vi "Initialize_main_SubVI.vi"() -> (0 "output cluster":T26 {"A/SPI - LiDAR"."SPI Configuration"."Frame Length" min=1 max=16})   [LabVIEW 2018]
uses:
  <vilib>/myRIO/Instrument Drivers/Onboard IO/DIO/typedefs/DIO Reference.ctl
  <vilib>/myRIO/Common/Instrument Driver Framework/Utilities/typedefs/myRIO Generic Hardware Reference.ctl
  <vilib>/myRIO/Common/Instrument Driver Framework/Utilities/typedefs/Hardware Version Enum.ctl
  <vilib>/myRIO/Common/Instrument Driver Framework/Utilities/typedefs/myRIO v1.0 Reference.ctl
  <vilib>/myRIO/Common/Instrument Driver Framework/Utilities/typedefs/Generic FPGA Reference.ctl
  <vilib>/myRIO/Common/Instrument Driver Framework/myRIO v1.0/DIO/typedefs/DIO Channels List.ctl
  <vilib>/myRIO/Common/Instrument Driver Framework/myRIO v1.0/DIO/typedefs/DIO Channels Enum.ctl
  <vilib>/myRIO/Instrument Drivers/Onboard IO/PWM/typedefs/PWM Reference.ctl
  <vilib>/myRIO/Common/Instrument Driver Framework/myRIO v1.0/PWM/typedefs/PWM Channels Enum.ctl
  <vilib>/myRIO/Instrument Drivers/Onboard IO/PWM/typedefs/PWM Configuration.ctl
  <vilib>/myRIO/Instrument Drivers/Onboard Devices/Accelerometer/typedefs/Accelerometer Reference.ctl
  <vilib>/myRIO/Common/Instrument Driver Framework/myRIO v1.0/Accelerometer/typedefs/Accelerometer Channels List.ctl
  <vilib>/myRIO/Common/Instrument Driver Framework/myRIO v1.0/Accelerometer/typedefs/Accelerometer Channels Enum.ctl
  <vilib>/myRIO/Instrument Drivers/Onboard IO/AI/typedefs/AI Reference.ctl
  <vilib>/myRIO/Common/Instrument Driver Framework/myRIO v1.0/AI/typedefs/AI Channels List.ctl
  <vilib>/myRIO/Common/Instrument Driver Framework/myRIO v1.0/AI/typedefs/AI Channels Enum.ctl
  <vilib>/myRIO/Common/Instrument Driver Framework/Utilities/typedefs/Analog Scaling Constants List.ctl
  <vilib>/myRIO/Common/Instrument Driver Framework/Utilities/typedefs/Analog Scaling Constants.ctl
  <vilib>/myRIO/Instrument Drivers/Onboard IO/SPI/typedefs/SPI Reference.ctl
  <vilib>/myRIO/Common/Instrument Driver Framework/myRIO v1.0/SPI/typedefs/SPI Channels Enum.ctl
  <vilib>/myRIO/Instrument Drivers/Onboard IO/SPI/typedefs/SPI Configuration.ctl
  <vilib>/myRIO/Common/Instrument Driver Framework/myRIO v1.0/SPI/typedefs/SPI Clock Phase.ctl
  <vilib>/myRIO/Common/Instrument Driver Framework/myRIO v1.0/SPI/typedefs/SPI Clock Polarity.ctl
  <vilib>/myRIO/Common/Instrument Driver Framework/myRIO v1.0/SPI/typedefs/SPI Data Direction.ctl
  <vilib>/myRIO/Common/Instrument Driver Framework/myRIO v1.0/SPI/typedefs/SPI Frame Length.ctl
  <vilib>/userdefined/High Color/nirio_resource_hc.ctl
  <vilib>/myRIO/Common/Instrument Driver Framework/myRIO v1.0/SPI/vis/myRIO v1.1 Open SPI.vi
  <vilib>/myRIO/Common/Instrument Driver Framework/myRIO v1.0/AI/vis/myRIO v1.1 Open AI.vi
  <vilib>/myRIO/Common/Instrument Driver Framework/myRIO v1.0/PWM/vis/myRIO v1.1 Open PWM.vi
  <vilib>/myRIO/Common/Instrument Driver Framework/myRIO v1.0/DIO/vis/myRIO v1.1 Open DIO.vi
  <vilib>/myRIO/Common/Instrument Driver Framework/myRIO v1.0/Accelerometer/vis/myRIO v1.1 Open Accelerometer.vi
  <vilib>/myRIO/Common/Instrument Driver Framework/Utilities/vis/Validate Channels.vi
  <vilib>/myRIO/Common/Instrument Driver Framework/myRIO v1.0/SPI/vis/myRIO v1.0 Reserve SPI.vi
  <vilib>/myRIO/Common/Instrument Driver Framework/myRIO v1.0/AI/vis/myRIO v1.0 Reserve AI.vi
  <vilib>/myRIO/Common/Instrument Driver Framework/myRIO v1.0/PWM/vis/myRIO v1.0 Reserve PWM.vi
  <vilib>/myRIO/Common/Instrument Driver Framework/myRIO v1.0/DIO/vis/myRIO v1.0 Reserve DIO.vi
  <vilib>/myRIO/Common/Instrument Driver Framework/myRIO v1.0/Accelerometer/vis/myRIO v1.0 Reserve Accelerometer.vi
  <vilib>/myRIO/Common/Instrument Driver Framework/myRIO v1.0/SPI/vis/myRIO v1.0 Build MUX Configuration SPI.vi
  <vilib>/myRIO/Common/Instrument Driver Framework/myRIO v1.0/Resource Manager/vis/myRIO v1.0 Reserve Channel List.vi
  <vilib>/myRIO/Common/Instrument Driver Framework/myRIO v1.0/AI/vis/myRIO v1.0 Build MUX Configuration AI.vi
  <vilib>/myRIO/Common/Instrument Driver Framework/myRIO v1.0/PWM/vis/myRIO v1.0 Build MUX Configuration PWM.vi
  <vilib>/myRIO/Common/Instrument Driver Framework/myRIO v1.0/DIO/vis/myRIO v1.0 Build MUX Configuration DIO.vi
  <vilib>/myRIO/Common/Instrument Driver Framework/myRIO v1.0/Accelerometer/vis/myRIO v1.0 Build MUX Configuration Accelerometer.vi
  <vilib>/myRIO/Common/Instrument Driver Framework/myRIO v1.0/Resource Manager/vis/myRIO v1.0 Create Configuration List.vi
  <vilib>/myRIO/Common/Instrument Driver Framework/myRIO v1.0/Resource Manager/vis/myRIO v1.0 Reserve Channel.vi
  <vilib>/myRIO/Common/Instrument Driver Framework/myRIO v1.0/Resource Manager/vis/myRIO v1.0 Unreserve Channel.vi
  <vilib>/myRIO/Common/Instrument Driver Framework/myRIO v1.0/Resource Manager/vis/myRIO v1.0 Build Mutex Name.vi
  <vilib>/Instr/_visa.llb/VISA Configure Serial Port (Instr).vi
  <vilib>/Utility/VariantDataType/GetNumericInfo.vi
  <vilib>/Utility/error.llb/Error Cluster From Error Code.vi
  <vilib>/myRIO/Common/Instrument Driver Framework/myRIO v1.0/myRIO v1.1 Open.vi
  <vilib>/myRIO/Common/Instrument Driver Framework/Utilities/vis/IO Manager.vi
  <vilib>/myRIO/Common/Instrument Driver Framework/Utilities/vis/Configuration Manager.vi
  <vilib>/myRIO/Common/Instrument Driver Framework/myRIO v1.0/Resource Manager/vis/myRIO v1.0 Configure IO.vi
  <vilib>/myRIO/Common/Instrument Driver Framework/myRIO v1.0/myRIO v1.0 Close.vi
  <vilib>/myRIO/Common/Instrument Driver Framework/myRIO v1.0/AI/vis/myRIO v1.0 Get Scaling Constants AI.vi
  <vilib>/myRIO/Common/Instrument Driver Framework/myRIO v1.0/Accelerometer/vis/myRIO v1.0 Get Scaling Constant Accelerometer.vi
  <vilib>/myRIO/Instrument Drivers/Onboard IO/PWM/vis/myRIO PWM Open.xnode
  <vilib>/myRIO/Instrument Drivers/Onboard IO/AI/vis/myRIO AI Open.xnode
  <vilib>/myRIO/Instrument Drivers/Onboard IO/DIO/vis/myRIO DIO Open.xnode
  <vilib>/myRIO/Instrument Drivers/Onboard Devices/Accelerometer/vis/myRIO Accelerometer Open.xnode
  <vilib>/myRIO/Instrument Drivers/Onboard IO/SPI/vis/myRIO SPI Open.xnode
  <vilib>/myRIO/Instrument Drivers/Onboard IO/DIO/DIO.lvlib
  <vilib>/myRIO/Instrument Drivers/Onboard IO/PWM/PWM.lvlib
  <vilib>/myRIO/Instrument Drivers/Onboard IO/AI/AI.lvlib
  <vilib>/myRIO/Instrument Drivers/Onboard Devices/Accelerometer/Accelerometer.lvlib
  <vilib>/myRIO/Instrument Drivers/Onboard IO/SPI/SPI.lvlib
panel:
  # "B/DIO0-Dir"
  # "DIR"
  # "B/DIO1-Enable for 1st Stepper"
  # "EN-1"
  # "B/DIO2-Enable for 2nd Stepper"
  # "EN-2"
  # "B/DIO3-Enable for 3nd Stepper"
  # "EN-3"
  # "B/DIO4-Endstop for 1st Stepper - Top"
  # "END-1-T"
  # "B/DIO11-Endstop for 1st Stepper - Bottom"
  # "END-1-B"
  # "B/DIO12-Endstop for 2nd Stepper - Top"
  # "END-2-T"
  # "B/DIO13-Endstop for 2nd Stepper - Bottom"
  # "END-2-B"
  # "B/DIO14-Endstop for 3rd Stepper - Top"
  # "END-3-T"
  # "B/DIO15-Endstop for 3rd Stepper - Bottom"
  # "END-3-B"
  # "Cooler"
  # "A/DIO0-Cooler"
  # "A/DIO1-Beacon drop (dio1)"
  # "Beacon drop"
  # "A/DIO2-Beacon drop (dio0)"
  # "Beacon drop"
  # "A/DIO3-QuickRelease (dio1)"
  # "QuickRelease"
  # "A/DIO4-QuickRelease (dio0)"
  # "QuickRelease"
  # "A/DIO11 - LiDAR Case selector"
  # "LiDAR CS"
  # "B/DIO8 - B_PWM0-Motor - Stepper"
  # "PWM-Step"
  # "B/DIO9 - B_PWM1- Drill motor"
  # "PWM-Drill"
  # "A/DIO8 - A_PWM0 - Servo_Roll"
  # "Gimbal_ROLL"
  # "A/DIO9 - A_PWM1 - Servo_Yaw"
  # "Gimbal_YAW"
  # "Accelerometer - X-axis"
  # "X-axis"
  # "Accelerometer - X-axis"
  # "Y-axis"
  # "B/AI0 - PWM from drone F3"
  # "Drone - F3 - Grounded"
  # "B/AI1 - PWM from drone F4"
  # "Drone - F4 - Drill gear"
  # "B/AI2 - PWM from drone F5"
  # "Drone - F5 - Beacon drop"
  # "B/AI3 - PWM from drone F6"
  # "Drone - F6 - Boost"
  # "A/AI0 - PWM from drone F8"
  # "Drone - F8 - Stepper"
  # "A/AI1 - Beacon Wiper"
  # "A/AI2 - QuickRelease Wiper"
  # "A/AI3 - Drill drawn current"
  # "A/SPI - LiDAR Distance measurement"
  # "B/UART - XBee Communication"
  # "A/UART - A3 GPS Coordinates"
  # "RIO - LEDs"
  # "RIO - LEDs"
types:
  T1 = typedef "DIO.lvlib/DIO Reference.ctl" = cluster{"myRIO Reference":T2, "DIO Channels List":T6}
  T2 = typedef "myRIO Generic Hardware Reference.ctl" = cluster{"myRIO Model":T3, "myRIO Hardware Reference":T4}
  T3 = typedef "Hardware Version Enum.ctl" = enum16{"Unknown", "myRIO-1900", "myRIO-1950", "roboRIO", "NI ELVIS RIO CM", "ELVIS III"}
  T4 = typedef "myRIO v1.0 Reference.ctl" = cluster{"Generic FPGA Reference":T5, "Allow multiple opens":bool}
  T5 = typedef "Generic FPGA Reference.ctl" = refnum<k20>
  T6 = typedef "DIO Channels List.ctl" = T7[]
  T7 = typedef "DIO Channels Enum.ctl" = enum16{"Not Connected", "C/DIO0", "C/DIO1", "C/DIO2", "C/DIO3", "C/DIO4", "C/DIO5", "C/DIO6", "C/DIO7", "A/DIO0", "A/DIO1", "A/DIO2", "A/DIO3", "A/DIO4", "A/DIO5", "A/DIO6", "A/DIO7", "A/DIO8", "A/DIO9", "A/DIO10", "A/DIO11", "A/DIO12", "A/DIO13", "A/DIO14", "A/DIO15", "A/DIO16", "A/DIO17", "A/DIO18", "A/DIO19", "B/DIO0", "B/DIO1", "B/DIO2", "B/DIO3", "B/DIO4", "B/DIO5", "B/DIO6", "B/DIO7", "B/DIO8", "B/DIO9", "B/DIO10", "B/DIO11", "B/DIO12", "B/DIO13", "B/DIO14", "B/DIO15", "B/DIO16", "B/DIO17", "B/DIO18", "B/DIO19", "LED0", "LED1", "LED2", "LED3", "Button0", "DIO/DIO0", "DIO/DIO1", "DIO/DIO2", "DIO/DIO3", "DIO/DIO4", "DIO/DIO5", "DIO/DIO6", "DIO/DIO7", "DIO/DIO8", "DIO/DIO9", "SPI/CS0", "SPI/CS1", "SPI/CS2", "SPI/CS3", "LED RADIO (Green)", "LED RADIO (Red)", "LED COMM (Green)", "LED COMM (Red)", "LED MODE (Green)", "LED MODE (Red)"}
  T8 = typedef "PWM.lvlib/PWM Reference.ctl" = cluster{"myRIO Reference":T2, "PWM Channels Enum":T9, "PWM Configuration":T10}
  T9 = typedef "PWM Channels Enum.ctl" = enum16{"Not Connected", "C/PWM0", "C/PWM1", "A/PWM0", "A/PWM1", "A/PWM2", "A/PWM3", "A/PWM4", "A/PWM5", "A/PWM6", "A/PWM7", "A/PWM8", "A/PWM9", "A/PWM10", "A/PWM11", "A/PWM12", "A/PWM13", "A/PWM14", "A/PWM15", "A/PWM16", "A/PWM17", "A/PWM18", "A/PWM19", "B/PWM0", "B/PWM1", "B/PWM2", "B/PWM3", "B/PWM4", "B/PWM5", "B/PWM6", "B/PWM7", "B/PWM8", "B/PWM9", "B/PWM10", "B/PWM11", "B/PWM12", "B/PWM13", "B/PWM14", "B/PWM15", "B/PWM16", "B/PWM17", "B/PWM18", "B/PWM19", "PWM/PWM0", "PWM/PWM1", "PWM/PWM2", "PWM/PWM3", "PWM/PWM4", "PWM/PWM5", "PWM/PWM6", "PWM/PWM7", "PWM/PWM8", "PWM/PWM9"}
  T10 = typedef "PWM.lvlib/PWM Configuration.ctl" = cluster{"Frequency":dbl, "Duty Cycle":dbl}
  T11 = typedef "Accelerometer.lvlib/Accelerometer Reference.ctl" = cluster{"myRIO Reference":T2, "Accelerometer Channels List":T12, "LSB Weight":dbl}
  T12 = typedef "Accelerometer Channels List.ctl" = T13[]
  T13 = typedef "Accelerometer Channels Enum.ctl" = enum16{"Not Connected", "X-Axis", "Y-Axis", "Z-Axis"}
  T14 = typedef "AI.lvlib/AI Reference.ctl" = cluster{"myRIO Reference":T2, "AI Channels List":T15, "AI Scaling Constants List":T17}
  T15 = typedef "AI Channels List.ctl" = T16[]
  T16 = typedef "AI Channels Enum.ctl" = enum16{"Not Connected", "AudioIn/Left", "AudioIn/Right", "C/AI0", "C/AI1", "A/AI0", "A/AI1", "A/AI2", "A/AI3", "A/AI4", "A/AI5", "A/AI6", "A/AI7", "B/AI0", "B/AI1", "B/AI2", "B/AI3", "B/AI4", "B/AI5", "B/AI6", "B/AI7", "AI/AI0", "AI/AI1", "AI/AI2", "AI/AI3", "A/AI0 (DIFF)", "A/AI1 (DIFF)", "A/AI2 (DIFF)", "A/AI3 (DIFF)", "B/AI0 (DIFF)", "B/AI1 (DIFF)", "B/AI2 (DIFF)", "B/AI3 (DIFF)"}
  T17 = typedef "Analog Scaling Constants List.ctl" = T18[]
  T18 = typedef "Analog Scaling Constants.ctl" = cluster{"LSB Weight (Volts)":dbl, "Offset (Volts)":dbl, "Signed?":bool}
  T19 = typedef "SPI.lvlib/SPI Reference.ctl" = cluster{"myRIO Reference":T2, "SPI Channels Enum":T20, "SPI Configuration":T21}
  T20 = typedef "SPI Channels Enum.ctl" = enum16{"Not Connected", "A/SPI", "B/SPI", "SPI/SPI"}
  T21 = typedef "SPI.lvlib/SPI Configuration.ctl" = cluster{"Frequency [Hz]":dbl, "Clock Phase":T22, "Clock Polarity":T23, "Data Direction":T24, "Frame Length":T25}
  T22 = typedef "SPI Clock Phase.ctl" = enum8{"Leading", "Trailing"}
  T23 = typedef "SPI Clock Polarity.ctl" = enum8{"Low", "High"}
  T24 = typedef "SPI Data Direction.ctl" = enum8{"Most significant bit first", "Least significant bit first"}
  T25 = typedef "SPI Frame Length.ctl" = u8
  T26 = cluster{"B/DIO0 - Stepper Direction":T1, "B/DIO1 - Stepper1 Enable":T1, "B/DIO2 - Stepper2 Enable":T1, "B/DIO3 - Stepper3 Enable":T1, "B/DIO4 - Endstop Stepper1 Top":T1, "B/DIO11 - Endstop Stepper1 Bund":T1, "B/DIO12 - Endstop Stepper2 Top":T1, "B/DIO13 - Endstop Stepper2 Bund":T1, "B/DIO14 - Endstop Stepper3 Top":T1, "B/DIO15 - Endstop Stepper3 Bund":T1, "A/DIO0 - Cooler":T1, "A/DIO1 - Beacon drop (dio1)":T1, "A/DIO2 - Beacon drop (dio0)":T1, "A/DIO3 - QuickRelease (dio1)":T1, "A/DIO4 - QuickRelease (dio0)":T1, "A/DIO11 - LiDAR SPI CS":T1, "B/PWM0 - Stepper":T8, "B/PWM1 - Drill":T8, "A/PWM0 - Servo_Roll":T8, "A/PWM1 - Servo_Yaw":T8, "Acc. X-axis":T11, "Acc. Y-axis":T11, "B/AI0 - Drone Grounded F3":T14, "B/AI1 - Drone Drill Gear F4":T14, "B/AI2 - Beacon Drop F5":T14, "B/AI3 - Drone Drill Boost F6":T14, "A/AI0 - Drone Stepper F8":T14, "A/AI1 - Beacon Wiper":T14, "A/AI2 - QuickRelease Wiper":T14, "A/AI3 - Drill Current":T14, "A/SPI - LiDAR":T19, "B/UART - XBee":refnum<visa-resource-name>, "A/UART - A3 GPS":refnum<visa-resource-name>, "RIO Flashing LEDs":T1}
  T27 = cluster{"DIO Ref Out":T1, "DIO Ref Out":T1, "DIO Ref Out":T1, "DIO Ref Out":T1, "DIO Ref Out":T1, "DIO Ref Out":T1, "DIO Ref Out":T1, "DIO Ref Out":T1, "DIO Ref Out":T1, "DIO Ref Out":T1, "DIO Ref Out":T1, "DIO Ref Out":T1, "DIO Ref Out":T1, "DIO Ref Out":T1, "DIO Ref Out":T1, "DIO Ref Out":T1, "PWM Ref Out":T8, "PWM Ref Out":T8, "PWM Ref Out":T8, "PWM Ref Out":T8, "Accelerometer Ref Out":T11, "Accelerometer Ref Out":T11, "AI Ref Out":T14, "AI Ref Out":T14, "AI Ref Out":T14, "AI Ref Out":T14, "AI Ref Out":T14, "AI Ref Out":T14, "AI Ref Out":T14, "AI Ref Out":T14, "SPI Ref Out":T19, "VISA resource name out":refnum<visa-resource-name>, "VISA resource name out":refnum<visa-resource-name>, "DIO Ref Out":T1}
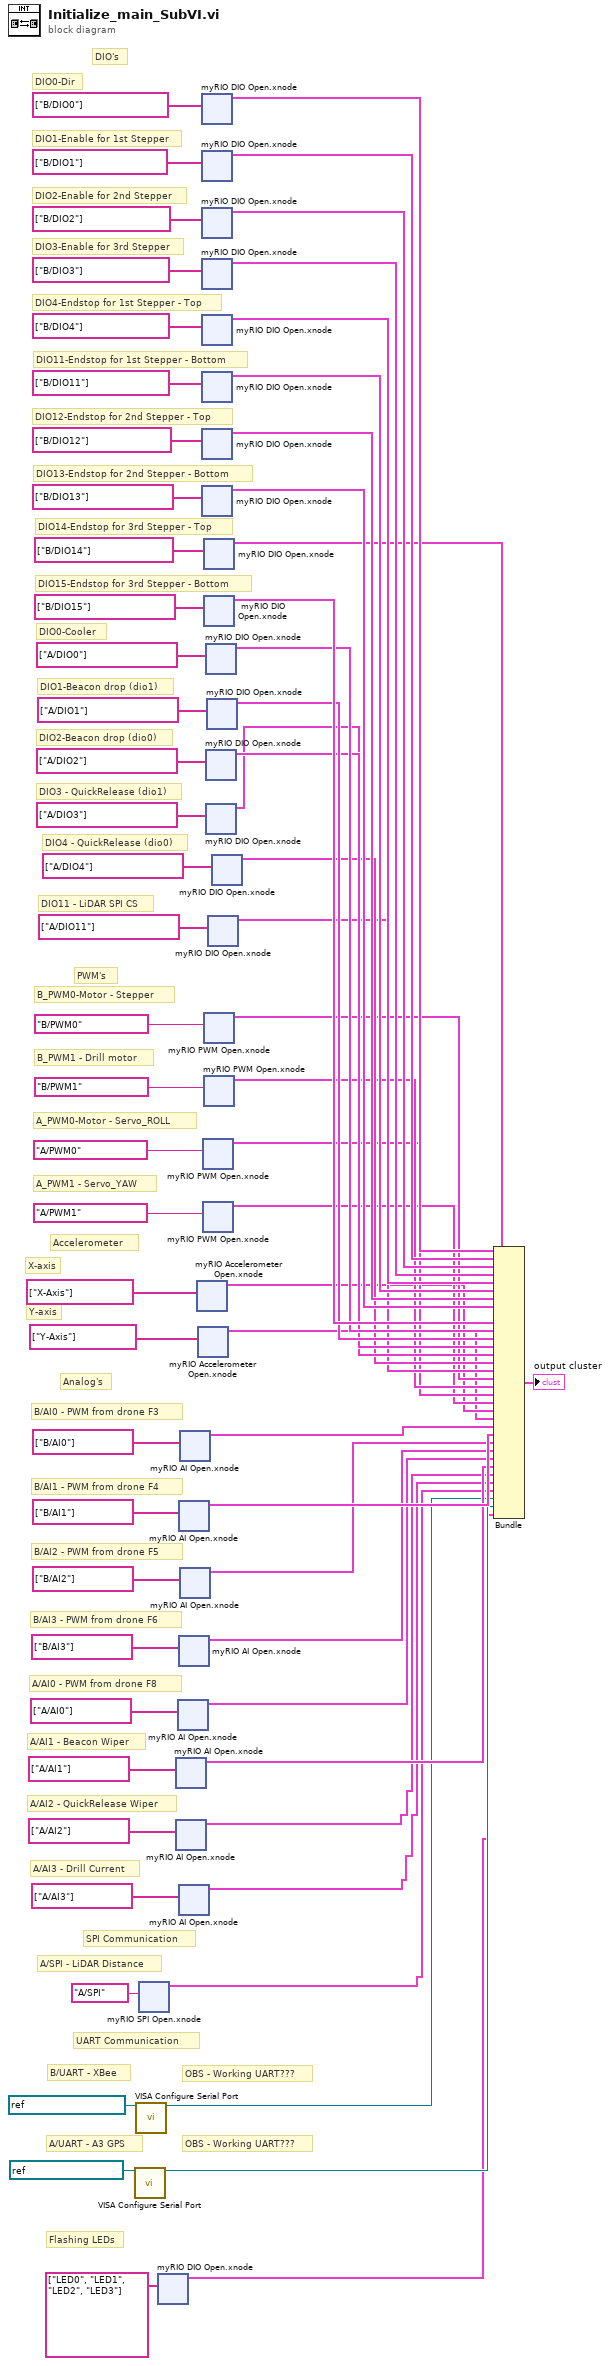
[diagram p0: block diagram]
diagram:
  # "OBS - Working UART???"
  # "OBS - Working UART???"
  # "Flashing LEDs"
  # "A/UART - A3 GPS"
  # "B/UART - XBee"
  # "A/SPI - LiDAR Distance"
  # "UART Communication"
  # "SPI Communication"
  # "A/AI3 - Drill Current"
  # "A/AI2 - QuickRelease Wiper"
  # "A/AI1 - Beacon Wiper"
  # "A_PWM1 - Servo_YAW"
  # "A_PWM0-Motor - Servo_ROLL"
  # "DIO11 - LiDAR SPI CS"
  # "DIO4 - QuickRelease (dio0)"
  # "DIO3 - QuickRelease (dio1)"
  # "DIO2-Beacon drop (dio0)"
  # "DIO1-Beacon drop (dio1)"
  # "Y-axis"
  # "DIO0-Cooler"
  # "A/AI0 - PWM from drone F8"
  # "B/AI3 - PWM from drone F6"
  # "DIO15-Endstop for 3rd Stepper - Bottom"
  # "DIO14-Endstop for 3rd Stepper - Top"
  # "DIO13-Endstop for 2nd Stepper - Bottom"
  # "DIO12-Endstop for 2nd Stepper - Top"
  # "DIO11-Endstop for 1st Stepper - Bottom"
  # "DIO4-Endstop for 1st Stepper - Top"
  # "Accelerometer"
  # "X-axis"
  # "DIO3-Enable for 3rd Stepper"
  # "DIO2-Enable for 2nd Stepper"
  # "DIO1-Enable for 1st Stepper"
  # "DIO0-Dir"
  # "Analog's"
  # "B/AI2 - PWM from drone F5"
  # "B/AI1 - PWM from drone F4"
  # "B/AI0 - PWM from drone F3"
  # "B_PWM1 - Drill motor"
  # "B_PWM0-Motor - Stepper"
  # "PWM's"
  # "DIO's"
  n1 = call-poly "VISA Configure Serial Port"("VISA resource name"=refnum<visa-resource-name> "ASRL1::INSTR") -> ("VISA resource name out"=w3:refnum<visa-resource-name>)  [unwired: 13 in, 1 out]
  n2 = call-poly "VISA Configure Serial Port"("VISA resource name"=refnum<visa-resource-name> "ASRL2::INSTR") -> ("VISA resource name out"=w4:refnum<visa-resource-name>)  [unwired: 13 in, 1 out]
  n3 = xnode "myRIO SPI Open.xnode"("Channel Name"=tag "A/SPI") -> ("SPI Ref Out"=w7:T19)  [unwired: 2 in, 1 out]
  n4 = xnode "myRIO DIO Open.xnode"("Channel Names"=tag[] ["LED0", "LED1", "LED2", "LED3"]) -> ("DIO Ref Out"=w2:T1)  [unwired: 2 in, 1 out]
  n5 = xnode "myRIO AI Open.xnode"("Channel Names"=tag[] ["A/AI1"]) -> ("AI Ref Out"=w11:T14)  [unwired: 2 in, 1 out]
  n6 = xnode "myRIO AI Open.xnode"("Channel Names"=tag[] ["A/AI2"]) -> ("AI Ref Out"=w10:T14)  [unwired: 2 in, 1 out]
  n7 = xnode "myRIO AI Open.xnode"("Channel Names"=tag[] ["A/AI0"]) -> ("AI Ref Out"=w12:T14)  [unwired: 2 in, 1 out]
  n8 = xnode "myRIO AI Open.xnode"("Channel Names"=tag[] ["B/AI1"]) -> ("AI Ref Out"=w15:T14)  [unwired: 2 in, 1 out]
  n9 = xnode "myRIO AI Open.xnode"("Channel Names"=tag[] ["B/AI3"]) -> ("AI Ref Out"=w13:T14)  [unwired: 2 in, 1 out]
  n10 = xnode "myRIO AI Open.xnode"("Channel Names"=tag[] ["A/AI3"]) -> ("AI Ref Out"=w9:T14)  [unwired: 2 in, 1 out]
  n11 = xnode "myRIO AI Open.xnode"("Channel Names"=tag[] ["B/AI0"]) -> ("AI Ref Out"=w16:T14)  [unwired: 2 in, 1 out]
  n12 = xnode "myRIO AI Open.xnode"("Channel Names"=tag[] ["B/AI2"]) -> ("AI Ref Out"=w14:T14)  [unwired: 2 in, 1 out]
  n13 = xnode "myRIO Accelerometer Open.xnode"("Channel Names"=tag[] ["X-Axis"]) -> ("Accelerometer Ref Out"=w21:T11)  [unwired: 2 in, 1 out]
  n14 = xnode "myRIO Accelerometer Open.xnode"("Channel Names"=tag[] ["Y-Axis"]) -> ("Accelerometer Ref Out"=w20:T11)  [unwired: 2 in, 1 out]
  n15 = xnode "myRIO DIO Open.xnode"("Channel Names"=tag[] ["B/DIO0"]) -> ("DIO Ref Out"=w53:T1)  [unwired: 2 in, 1 out]
  n16 = xnode "myRIO DIO Open.xnode"("Channel Names"=tag[] ["B/DIO1"]) -> ("DIO Ref Out"=w52:T1)  [unwired: 2 in, 1 out]
  n17 = xnode "myRIO DIO Open.xnode"("Channel Names"=tag[] ["B/DIO2"]) -> ("DIO Ref Out"=w51:T1)  [unwired: 2 in, 1 out]
  n18 = xnode "myRIO DIO Open.xnode"("Channel Names"=tag[] ["B/DIO3"]) -> ("DIO Ref Out"=w50:T1)  [unwired: 2 in, 1 out]
  n19 = xnode "myRIO DIO Open.xnode"("Channel Names"=tag[] ["B/DIO4"]) -> ("DIO Ref Out"=w49:T1)  [unwired: 2 in, 1 out]
  n20 = xnode "myRIO DIO Open.xnode"("Channel Names"=tag[] ["B/DIO11"]) -> ("DIO Ref Out"=w48:T1)  [unwired: 2 in, 1 out]
  n21 = xnode "myRIO DIO Open.xnode"("Channel Names"=tag[] ["B/DIO12"]) -> ("DIO Ref Out"=w47:T1)  [unwired: 2 in, 1 out]
  n22 = xnode "myRIO DIO Open.xnode"("Channel Names"=tag[] ["B/DIO13"]) -> ("DIO Ref Out"=w46:T1)  [unwired: 2 in, 1 out]
  n23 = xnode "myRIO PWM Open.xnode"("Channel Name"=tag "A/PWM0") -> ("PWM Ref Out"=w23:T8)  [unwired: 2 in, 1 out]
  n24 = xnode "myRIO PWM Open.xnode"("Channel Name"=tag "A/PWM1") -> ("PWM Ref Out"=w22:T8)  [unwired: 2 in, 1 out]
  n25 = xnode "myRIO DIO Open.xnode"("Channel Names"=tag[] ["B/DIO14"]) -> ("DIO Ref Out"=w45:T1)  [unwired: 2 in, 1 out]
  n26 = xnode "myRIO DIO Open.xnode"("Channel Names"=tag[] ["B/DIO15"]) -> ("DIO Ref Out"=w44:T1)  [unwired: 2 in, 1 out]
  n27 = xnode "myRIO PWM Open.xnode"("Channel Name"=tag "B/PWM0") -> ("PWM Ref Out"=w25:T8)  [unwired: 2 in, 1 out]
  n28 = xnode "myRIO PWM Open.xnode"("Channel Name"=tag "B/PWM1") -> ("PWM Ref Out"=w24:T8)  [unwired: 2 in, 1 out]
  n29 = xnode "myRIO DIO Open.xnode"("Channel Names"=tag[] ["A/DIO0"]) -> ("DIO Ref Out"=w36:T1)  [unwired: 2 in, 1 out]
  n30 = xnode "myRIO DIO Open.xnode"("Channel Names"=tag[] ["A/DIO2"]) -> ("DIO Ref Out"=w34:T1)  [unwired: 2 in, 1 out]
  n31 = xnode "myRIO DIO Open.xnode"("Channel Names"=tag[] ["A/DIO3"]) -> ("DIO Ref Out"=w30:T1)  [unwired: 2 in, 1 out]
  n32 = xnode "myRIO DIO Open.xnode"("Channel Names"=tag[] ["A/DIO1"]) -> ("DIO Ref Out"=w35:T1)  [unwired: 2 in, 1 out]
  n33 = xnode "myRIO DIO Open.xnode"("Channel Names"=tag[] ["A/DIO11"]) -> ("DIO Ref Out"=w28:T1)  [unwired: 2 in, 1 out]
  n34 = xnode "myRIO DIO Open.xnode"("Channel Names"=tag[] ["A/DIO4"]) -> ("DIO Ref Out"=w29:T1)  [unwired: 2 in, 1 out]
  n35 = Bundle("DIO Ref Out"=w53, "DIO Ref Out"=w52, "DIO Ref Out"=w51, "DIO Ref Out"=w50, "DIO Ref Out"=w49, "DIO Ref Out"=w48, "DIO Ref Out"=w47, "DIO Ref Out"=w46, "DIO Ref Out"=w45, "DIO Ref Out"=w44, "DIO Ref Out"=w36, "DIO Ref Out"=w35, "DIO Ref Out"=w34, "DIO Ref Out"=w30, "DIO Ref Out"=w29, "DIO Ref Out"=w28, "PWM Ref Out"=w25, "PWM Ref Out"=w24, "PWM Ref Out"=w23, "PWM Ref Out"=w22, "Accelerometer Ref Out"=w21, "Accelerometer Ref Out"=w20, "AI Ref Out"=w16, "AI Ref Out"=w15, "AI Ref Out"=w14, "AI Ref Out"=w13, "AI Ref Out"=w12, "AI Ref Out"=w11, "AI Ref Out"=w10, "AI Ref Out"=w9, "SPI Ref Out"=w7, "VISA resource name out"=w4, "VISA resource name out"=w3, "DIO Ref Out"=w2) -> (→"output cluster":T27)  [unwired: 1 in]
